vi "Configure CSV.vi"(8 "error in (no error)":errorcluster, 11 "Settings IN":T1) -> (0 "error out":errorcluster, 3 "Settings OUT":T1)   [LabVIEW 2017, in "Acquisition.lvlib"]
doc: "Configure the hardware."
uses:
  Acquisition.lvlib
  Acquisition Settings.ctl
  Acquisition State.ctl
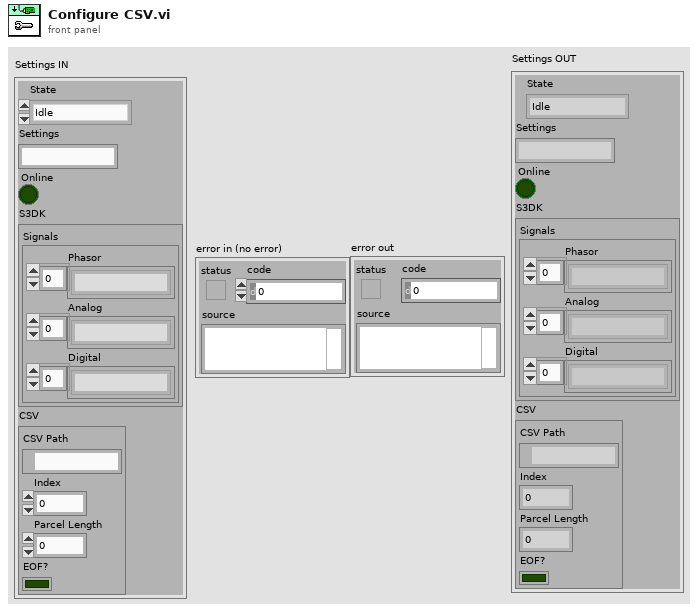
[diagram p1: front panel]
types:
  T1 = typedef "Acquisition.lvlib/Acquisition Settings.ctl" = cluster{"State":T2, "Settings":string, "Online":bool, "S3DK":cluster{"Signals":cluster{"Phasor":string[], "Analog":string[], "Digital":string[]}}, "CSV":cluster{"CSV Path":path, "Index":i32, "Parcel Length":i32, "EOF?":bool}}
  T2 = typedef "Acquisition.lvlib/Acquisition State.ctl" = enum16{"Idle", "Idle S3DK", "Acquiring S3DK", "Idle CSV", "Acquiring CSV"}
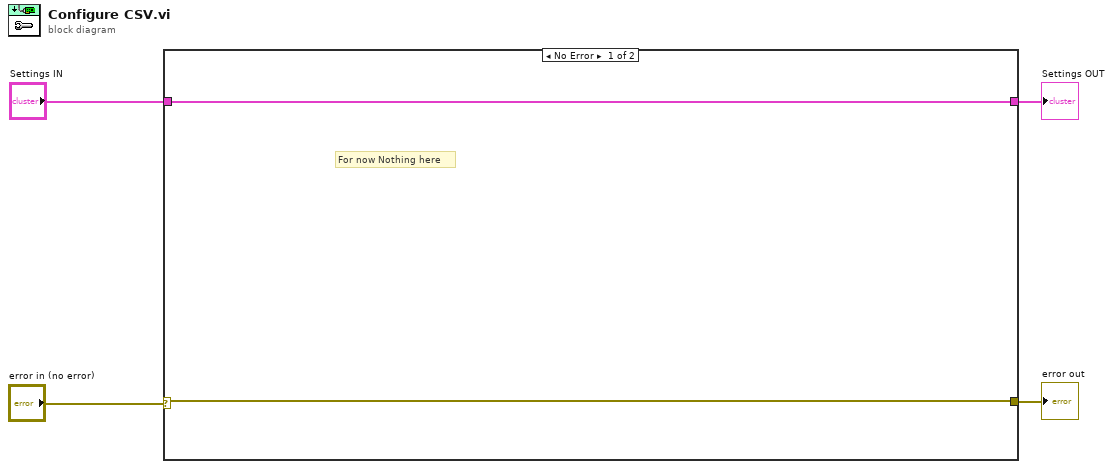
[diagram p0: block diagram]
diagram:
  n1 = case shown="No Error" "error in (no error)" {
    selector: "error in (no error)" -> [w6 w7]
    tunnel: [w6 w7] -> w3
    tunnel: "Settings IN" -> [w5 w8]
    tunnel: [w5 w8] -> w1
    frame No Error {
      # "For now Nothing here"
    }
    frame Error {
    }
  }
  "Settings OUT" <- w1
  "error out" <- w3
